vi "_dpo3014_read.vi"(4 "error in (no error)":errorcluster, 5 "Number of points":u32, 6 "Channel":u16(ring) items=["Ch1", "Ch2", "Ch3", "Ch4"], 7 "Oscilloscope Address":refnum<visa-resource-name>="USB0::0x0699::0x0373::C010680::INSTR") -> (0 "error out":errorcluster, 1 "Channel  Graph":dbl[](graph), 2 "Channel Data":dbl[](array[numeric]), 3 "Oscilloscope Address Out":refnum<visa-resource-name>="USB0::0x0699::0x0373::C010680::INSTR")   [LabVIEW 2013]
panel:
  out "Raw data":string
  out "Number of requests made":u32
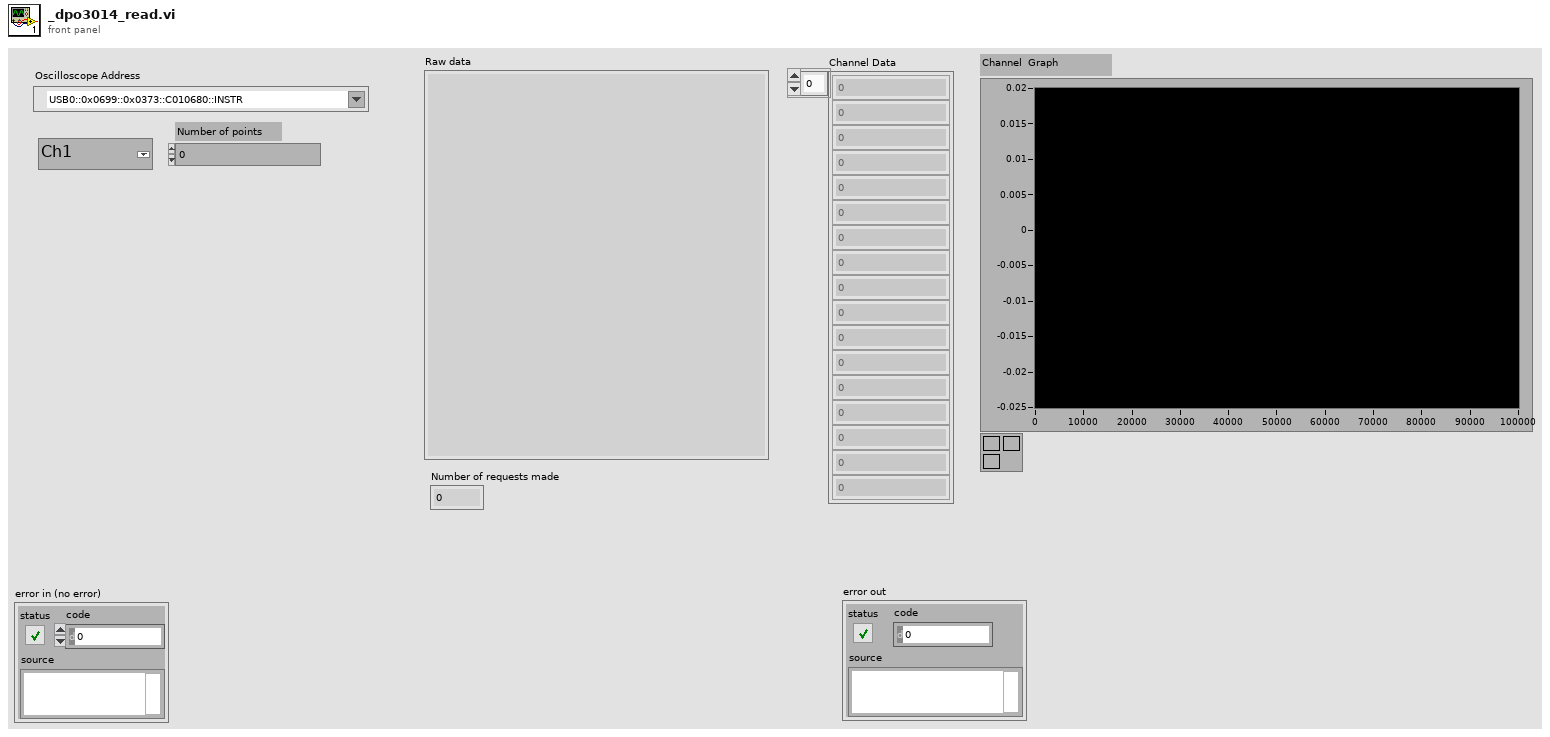
[diagram p1: front panel]
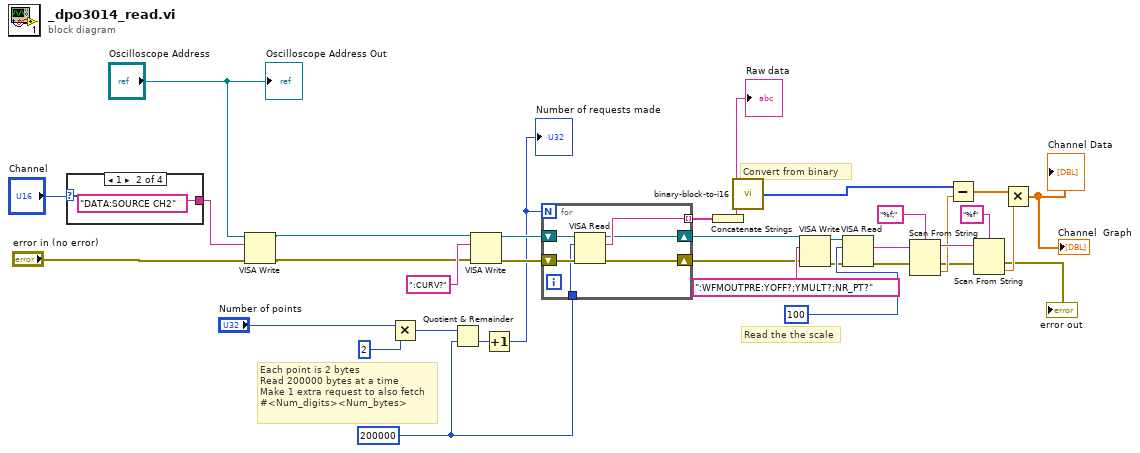
[diagram p0: block diagram]
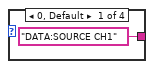
[diagram p2: hidden frame]
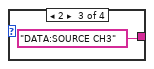
[diagram p3: hidden frame]
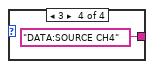
[diagram p4: hidden frame]
diagram:
  w7 = u32 200000 ("y")
  # "Each point is 2 bytes\nRead 200000 bytes at a time\nMake 1 extra request to also fetch\n#<Num_digits><Num_bytes>"
  # "Convert from binary"
  # "Read the the scale"
  n1 = case shown="1" "Channel" {
    tunnel: ["DATA:SOURCE CH1" "DATA:SOURCE CH2" "DATA:SOURCE CH3" "DATA:SOURCE CH4"] -> w35
    frame 0, Default {
    }
    frame 1 {
    }
    frame 2 {
    }
    frame 3 {
    }
  }
  n2 = VISA Write(VISA resource name="Oscilloscope Address", write buffer=w35, error in (no error)="error in (no error)") -> (VISA resource name out=w1:refnum<visa-resource-name>, error out=w2:errorcluster)  [unwired: 1 out]
  n3 = Multiply(x="Number of points", y=u32 2) -> (x*y=w10:u32)
  n4 = Quotient & Remainder(x=w10, y=w7) -> (floor(x/y)=w9:u32)  [unwired: 1 out]
  n5 = VISA Write(VISA resource name=w1, write buffer=":CURV?", error in (no error)=w2) -> (VISA resource name out=w21:refnum<visa-resource-name>, error out=w17:errorcluster)  [unwired: 1 out]
  n6 = Increment(x=w9) -> (x+1=w8:u32)
  "Number of requests made" <- w8
  n7 = for {
    N: w8 -> [_]
    shift-right: [w40] -> w16
    shift-left: w17 -> [w44]
    tunnel: w7 -> [w43]
    tunnel: [w42] -> w6 mode=indexing
    shift-right: [w41] -> w4
    shift-left: w21 -> [w45]
    n8 = VISA Read(VISA resource name=w45, byte count=w43, error in (no error)=w44) -> (VISA resource name out=w41:refnum<visa-resource-name>, read buffer=w42:string, error out=w40:errorcluster)  [unwired: 1 out]
  }
  n9 = Concatenate Strings(w6) -> (w5:string)
  "Raw data" <- w5
  n10 = call "binary-block-to-i16.vi"("Binary Block"=w5) -> ("i16 Array"=w29:i32[])
  n11 = VISA Write(VISA resource name=w4, write buffer=":WFMOUTPRE:YOFF?;YMULT?;NR_PT?", error in (no error)=w16) -> (VISA resource name out=w23:refnum<visa-resource-name>, error out=w15:errorcluster)  [unwired: 1 out]
  n12 = VISA Read(VISA resource name=w23, byte count=u32 100, error in (no error)=w15) -> (read buffer=w26:string, error out=w14:errorcluster)  [unwired: 2 out]
  n13 = Scan From String(format string="%f;", input string=w26, error in=w14) -> (remaining string=w31:string, error out=w13:errorcluster, output 1=w28:dbl)  [unwired: 2 in, 1 out]
  n14 = Subtract(x=w29, y=w28) -> (x-y=w33:dbl[])
  n15 = Scan From String(format string="%f", input string=w31, error in=w13) -> (error out=→"error out":errorcluster, output 1=w32:dbl)  [unwired: 2 in, 2 out]
  n16 = Multiply(x=w33, y=w32) -> (x*y=→"Channel Data" →"Channel  Graph":dbl[])
  "Oscilloscope Address Out" <- "Oscilloscope Address"
